vi "Locate Cornea.vi"(7 "error in":errorcluster) -> (20 "Matches (Pattern Matching 1)":T2(array[cluster]) {"Bounding Box"."y" format="%.2f"; "Bounding Box"."x" format="%.2f"; "Position"."y" format="%.2f"; "Position"."x" format="%.2f"; "Score" format="%.2f"; "Scale" format="%.2f"; "Angle" format="%.2f"}, 21 "Calibrated Matches (Pattern Matching 1)":T2(array[cluster]) {"Bounding Box"."y" format="%.2f"; "Bounding Box"."x" format="%.2f"; "Position"."y" format="%.2f"; "Position"."x" format="%.2f"; "Score" format="%.2f"; "Scale" format="%.2f"; "Angle" format="%.2f"}, 27 "error out":errorcluster)   [LabVIEW 2014]
uses:
  <vilib>/vision/NI_Vision_Development_Module.lvlib
panel:
  in  "File Path":path
  out "Image Out":T1(plugin-control)
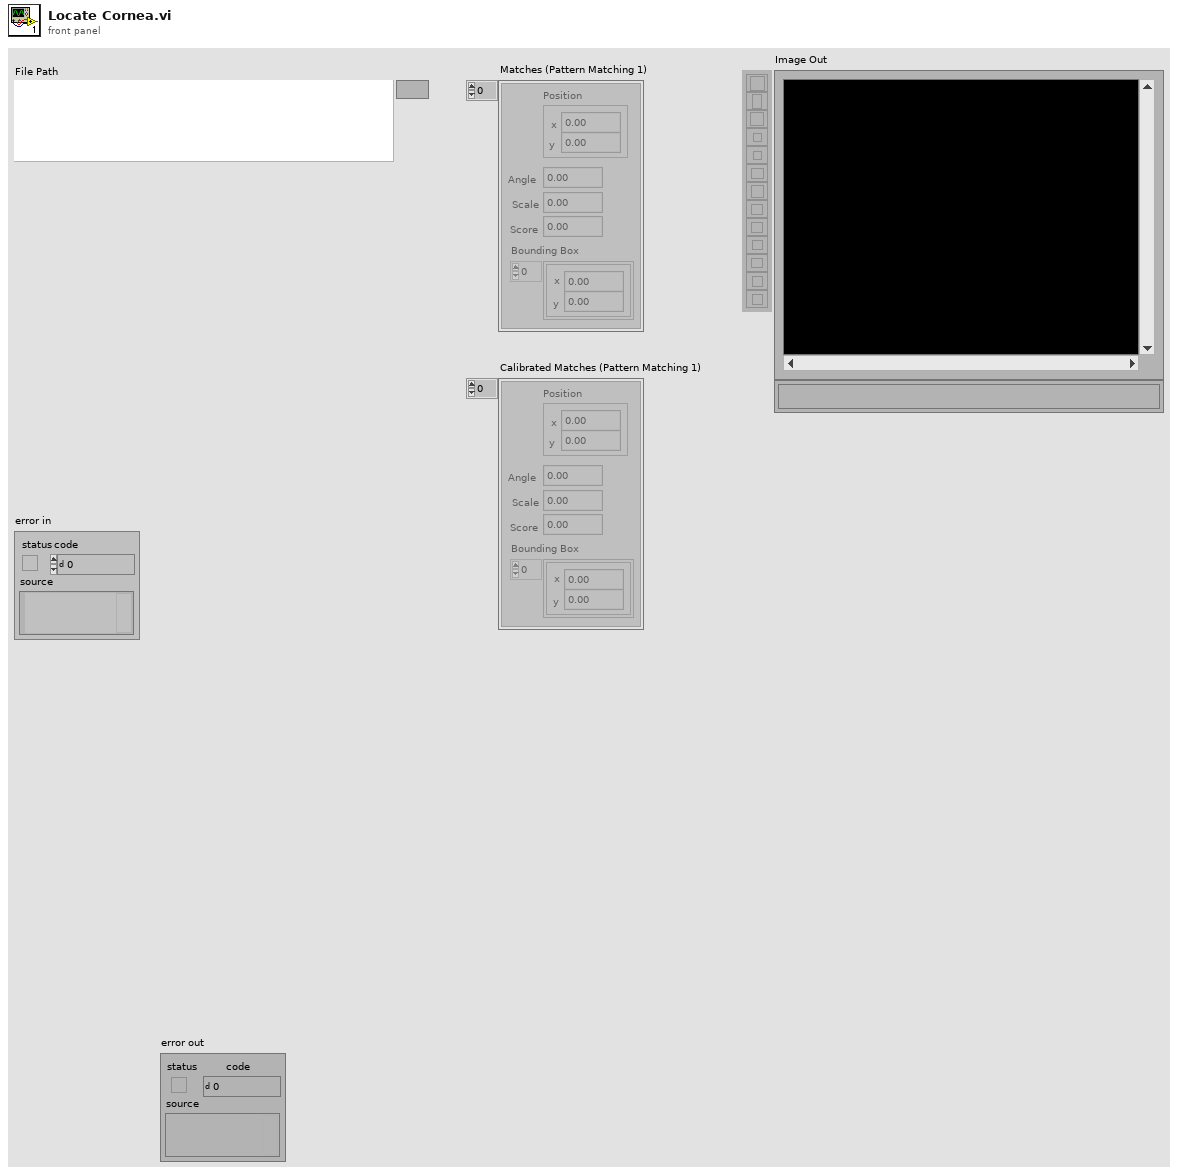
[diagram p1: front panel]
types:
  T1 = typedef "IMAQ Image.ctl" = refnum<image>
  T2 = cluster{"Position":cluster{"x":sgl, "y":sgl}, "Angle":sgl, "Scale":sgl, "Score":sgl, "Bounding Box":cluster{"x":sgl, "y":sgl}[]}[]
  T3 = cluster{"Number of Matches Requested":i32, "Minimum Match Score":sgl, "Angle Ranges":cluster{"Start Angle":sgl, "End Angle":sgl}[]}
  T4 = cluster{"Global Rectangle":i32[], "Contours":cluster{"ID":enum32{"External", "Internal"}, "Type":u32, "Coordinates":i32[]}[]}
  T5 = typedef "Image Type" = u32
  T6 = cluster{"histogram":u32[], "Minimal Value":sgl, "Maximal Value":sgl, "Starting Value":sgl, "Interval Width":sgl, "Mean Value":sgl, "Standard  Variation":sgl, "Area (pixels)":i32}
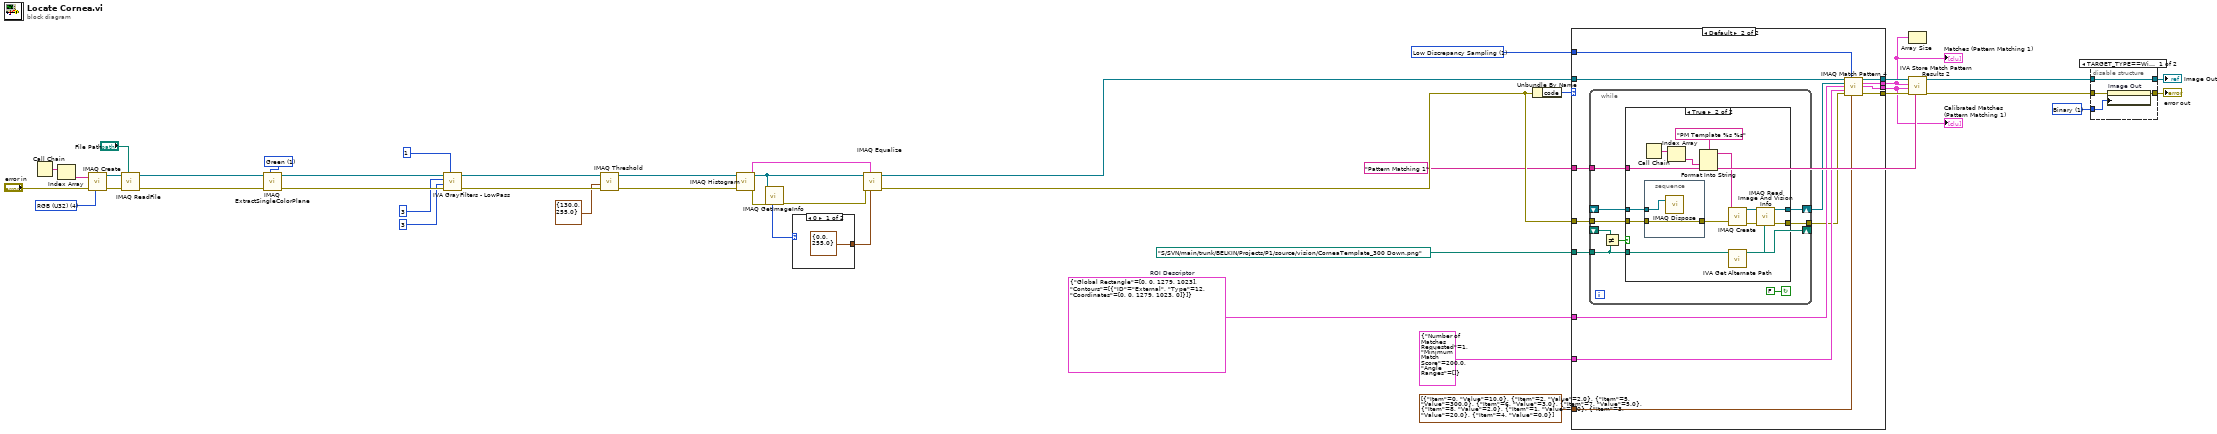
[diagram p0: block diagram]
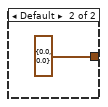
[diagram p5: hidden frame]
diagram:
  w1 = u32 1 items=["Grayscale", "Binary", "Gradient", "Rainbow", "Temperature", "User Defined"] ("Palette")
  w11 = 1 items=["All", "Low Discrepancy Sampling", "Grayscale Value Pyramid", "Gradients Pyramid"] ("Algorithm")
  w7 = "Pattern Matching 1" ("Step Name")
  w10 = T4 {"Global Rectangle"=[0, 0, 1279, 1023], "Contours"=[{"ID"=enum."External", "Type"=12, "Coordinates"=[0, 0, 1279, 1023, 0]}]}  # ROI Descriptor
  w35 = 1 items=["Red", "Green", "Blue", "Hue", "Saturation", "Luminance", "Value", "Intensity"] ("Color Plane")
  w36 = T5 4 items=["Grayscale (U8)", "Grayscale (I16)", "Grayscale (SGL)", "Complex (CSG)", "RGB (U32)", "HSL (U32)", "RGB (U64)", "Grayscale (U16)"] ("Image Type")
  n1 = Call Chain() -> (call chain=w39:string[])
  n2 = Index Array(array=w39) -> (element=w38:string)  [unwired: 1 in]
  n3 = call "IMAQ Create"("Image Name"=w38, "Image Type"=w36, "error in (no error)"="error in") -> ("New Image"=w42:T1, "error out"=w41:errorcluster)  [unwired: 1 in, 1 out]
  n4 = call "IMAQ ReadFile"("File Path"="File Path", "error in (no error)"=w41, "Image"=w42) -> ("error out"=w43:errorcluster, "Image Out"=w34:T1)  [unwired: 2 in, 5 out]
  n5 = call "IMAQ ExtractSingleColorPlane"("Color Plane"=w35, "error in (no error)"=w43, "Image Src"=w34) -> ("error out"=w33:errorcluster, "Image Dst Out"=w32:T1)  [unwired: 1 in, 6 out]
  n6 = call <vilib>:"IVA GrayFilters - LowPass.vi"("Tolerance"=1, "error in"=w33, "Filter size Y"=3, "Filter size X"=3, "Image In"=w32) -> ("error out"=w31:errorcluster, "Image Out"=w26:T1)  [unwired: 5 out]
  n7 = call "IMAQ Threshold"("error in (no error)"=w31, "Range"=cluster{"Lower value":sgl, "Upper value":sgl} {"Lower value"=130.0, "Upper value"=255.0}, "Image Src"=w26) -> ("error out"=w25:errorcluster, "Image Dst Out"=w21:T1)  [unwired: 3 in, 4 out]
  n8 = call "IMAQ Histogram"("error in (no error)"=w25, "Image"=w21) -> ("error out"=w20:errorcluster, "Histogram Report"=w23:T6)  [unwired: 3 in, 5 out]
  n9 = call "IMAQ GetImageInfo"("error in (no error)"=w20, "Image"=w21) -> ("error out"=w19:errorcluster, "Image Type"=w22:T5)  [unwired: 8 out]
  n10 = case shown="0" w22 {
    tunnel: [cluster{"Minimum":sgl, "Maximum":sgl} {"Minimum"=0.0, "Maximum"=255.0} ("Range") cluster{"Minimum":sgl, "Maximum":sgl} {"Minimum"=0.0, "Maximum"=0.0} ("Range")] -> w18
    frame 0 {
    }
    frame Default {
    }
  }
  n11 = call "IMAQ Equalize"("Range"=w18, "Histogram Report"=w23, "error in (no error)"=w19, "Image Src"=w21) -> ("error out"=w24:errorcluster, "Image Dst Out"=w16:T1)  [unwired: 2 in, 4 out]
  n12 = Unbundle By Name(w24) -> ("code"=w12:i32)
  n13 = case shown="Default" w12 {
    tunnel: path "S:/SVN/main/trunk/BELKIN/Projects/P1/source/vision/CorneaTemplate_300 Down.png" ("Template File Path") -> [_ w60]
    tunnel: w24 -> [_ w59]
    tunnel: w16 -> [w46 w54]
    tunnel: [_ w55] -> w15
    tunnel: [_ w56] -> w6
    tunnel: [w46 w53] -> w13
    tunnel: w7 -> [_ w58]
    tunnel: w11 -> [_ w52]
    tunnel: w10 -> [_ w51]
    tunnel: T3 {"Number of Matches Requested"=1, "Minimum Match Score"=200.0, "Angle Ranges"=[]} ("Parameters") -> [_ w50]
    tunnel: cluster{"Item":u16, "Value":dbl}[] [{"Item"=0, "Value"=10.0}, {"Item"=2, "Value"=2.0}, {"Item"=5, "Value"=300.0}, {"Item"=6, "Value"=3.0}, {"Item"=7, "Value"=5.0}, {"Item"=8, "Value"=2.0}, {"Item"=1, "Value"=1.0}, {"Item"=3, "Value"=20.0}, {"Item"=4, "Value"=0.0}] ("Advanced Options") -> [_ w48]
    tunnel: [_ w47] -> w5
    frame -1074396199, -1074396198 {
      # "Discard Coordinate System Error"
    }
    frame Default {
      n14 = while {
        shift-right: [w69] -> w57
        shift-left: _ -> [w68]
        tunnel: [w66] -> w49
        tunnel: w59 -> [w65]
        tunnel: w60 -> [w62]
        tunnel: w58 -> [w64]
        shift-right: [w62] -> _
        shift-left: _ -> [w63]
        stop <- FALSE continue-if-true
        n15 = Not Equal?(x=w63, y=w62) -> (x != y?=w61:bool)
        n16 = case shown="True" w61 {
          tunnel: [w71 w83] -> w69
          tunnel: w68 -> [w71 w74]
          tunnel: [w70 w80] -> w66
          tunnel: w65 -> [w70 w73]
          tunnel: w62 -> [_ w76]
          tunnel: w64 -> [_ w77]
          frame False {
          }
          frame True {
            n17 = stacked-sequence {
              tunnel: w74 -> [w87]
              tunnel: w73 -> [w86]
              tunnel: [w86] -> w72
              frame #0 {
                n18 = call "IMAQ Dispose"("Image"=w87) -> ()  [unwired: 2 in, 4 out]
              }
            }
            n19 = Call Chain() -> (call chain=w79:string[])
            n20 = Index Array(array=w79) -> (element=w78:string)  [unwired: 1 in]
            n21 = Format Into String(format string="PM Template %s %s" ("Image Name"), w78, w77) -> (resulting string=w85:string)  [unwired: 2 in, 1 out]
            n22 = call "IMAQ Create"("Image Name"=w85, "error in (no error)"=w72) -> ("New Image"=w82:T1, "error out"=w81:errorcluster)  [unwired: 2 in, 1 out]
            n23 = call <vilib>:"IVA Get Alternate Path.vi"("Path In"=w76) -> ("Path Out"=w75:path)  [unwired: 10 out]
            n24 = call "IMAQ Read Image And Vision Info"("File Path"=w75, "error in (no error)"=w81, "Image"=w82) -> ("error out"=w80:errorcluster, "Image Out"=w83:T1)  [unwired: 1 in, 6 out]
          }
        }
      }
      n25 = call "IMAQ Match Pattern 4"("Image"=w54, "Algorithm"=w52, "Template Image"=w57, "ROI Descriptor"=w51, "Parameters"=w50, "error in (no error)"=w49, "Advanced Options"=w48) -> ("Image (duplicate)"=w53:T1, "Matches (pixel)"=w56:T2, "Matches (real-world)"=w47:T2, "error out"=w55:errorcluster)  [unwired: 4 in, 1 out]
    }
  }
  "Matches (Pattern Matching 1)" <- w6
  "Calibrated Matches (Pattern Matching 1)" <- w5
  n26 = Array Size(array=w6) -> ()  [unwired: 1 out]
  n27 = call <vilib>:"IVA Store Match Pattern Results 2.vi"("Step Name"=w7, "error in (no error)"=w15, "Matches (real-world)"=w5, "Matches (pixel)"=w6, "Image in"=w13) -> ("error out"=w14:errorcluster, "Image dup"=w3:T1)  [unwired: 1 in, 4 out]
  n28 = disable-structure "Conditional Disable Structure" shown="TARGET_TYPE==Windows" {
    disable-tunnel: w14 -> [w91 w92]
    disable-tunnel: [w90 w92] -> w4
    disable-tunnel: w3 -> [w89 w93]
    disable-tunnel: [w89 w93] -> w2
    disable-tunnel: w1 -> [w88 _]
    frame condition #0 (active) {
      n29 = property on="Image Out" class="ImageControl"(error in=w91, "Palette:Palette Type"=w88) -> (error out=w90:errorcluster)  [unwired: 1 in, 1 out]
    }
    frame condition #1 {
    }
  }
  "error out" <- w4
  "Image Out" <- w2
